vi "RPC Method NIMeasurementServices_RegistryService_UnregisterService.vi"(8 "error in (no error)":errorcluster, 10 "Request Data":T2, 11 "gRPC Client in":refnum<class "Discovery_client.lvclass">) -> (0 "error out":errorcluster, 2 "Response Data":T1, 3 "gRPC Client out":refnum<class "Discovery_client.lvclass">)   [LabVIEW 2019, in "Discovery_client.lvlib" / "Discovery_client.lvclass"]
uses:
  Discovery_client.lvclass
  RPC Messages/NIMeasurementServices_UnregisterServiceRequest/NIMeasurementServices_UnregisterServiceRequest_Data.ctl
  RPC Messages/NIMeasurementServices_UnregisterServiceResponse/NIMeasurementServices_UnregisterServiceResponse_Data.ctl
  Discovery_client.lvclass/Discovery_client.ctl
  fa22ca14-33b2-4bc3-8699-3f27c9b27c9c.vi
  <vilib>/gRPC/LabVIEW gRPC Library/Server API/Server/Get Server DLL Path.vi
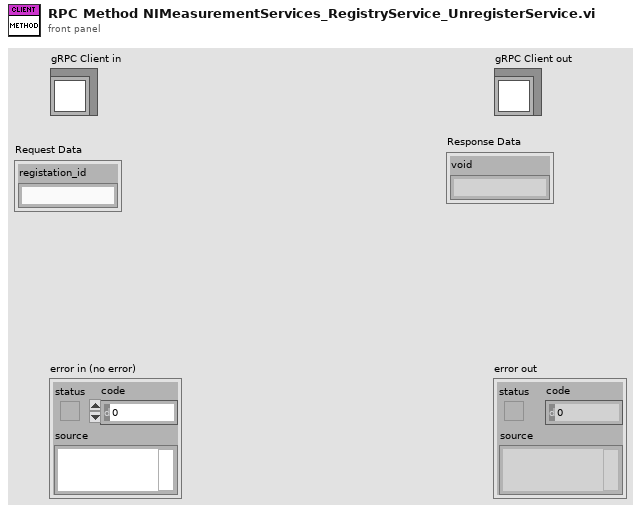
[diagram p1: front panel]
types:
  T1 = typedef "Discovery_client.lvlib/Discovery_client.lvclass/NIMeasurementServices_UnregisterServiceResponse_Data.ctl" = cluster{"void":string}
  T2 = typedef "Discovery_client.lvlib/Discovery_client.lvclass/NIMeasurementServices_UnregisterServiceRequest_Data.ctl" = cluster{"registation_id":string}
  T3 = typedef "gprc-lvsupport-release.lvlib/grpcId.ctl" = u64
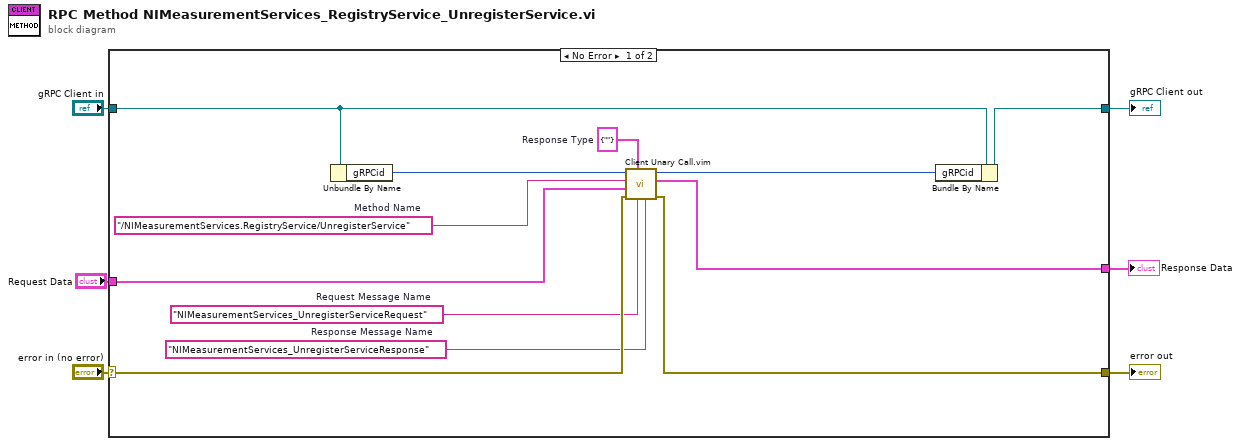
[diagram p0: block diagram]
diagram:
  n1 = case shown="No Error" "error in (no error)" {
    selector: "error in (no error)" -> [w14 w20]
    tunnel: [w13 w20] -> w5
    tunnel: [w15 w19] -> w3
    tunnel: "gRPC Client in" -> [w17 w19]
    tunnel: "Request Data" -> [w11 _]
    tunnel: [w10 _] -> w1
    frame No Error {
      w7 = "NIMeasurementServices_UnregisterServiceResponse"  # Response Message Name
      w8 = "NIMeasurementServices_UnregisterServiceRequest"  # Request Message Name
      w9 = T1 {"void"=""}  # Response Type
      w12 = "/NIMeasurementServices.RegistryService/UnregisterService"  # Method Name
      n2 = Unbundle By Name(w17) -> ("gRPCid"=w18:T3)
      n3 = call "Client Unary Call.vim"("Response Message Name"=w7, "Request Message Name"=w8, "Response Type"=w9, "error in (no error)"=w14, "Request Data"=w11, "Method Name"=w12, "Client Ref"=w18) -> ("error out"=w13:errorcluster, "Response Data"=w10:T1, "Client Ref Out"=w16:u64)  [unwired: 2 in]
      n4 = Bundle By Name(cluster=w17, "gRPCid"=w16) -> (w15:refnum<class "Discovery_client.lvclass">)
    }
    frame Error {
    }
  }
  "error out" <- w5
  "gRPC Client out" <- w3
  "Response Data" <- w1
